vi "Find EXE Root.vi"(10 "Path":path) -> (2 "Location of EXE":path)   [LabVIEW 2026, in "Controller Actor.lvlib" / "Controller.lvclass"]
uses:
  Controller.lvclass
  Controller.lvclass/Controller.ctl
  <userlib>/_OpenG.lib/file/file.llb/Strip Path Extension - String__ogtk.vi
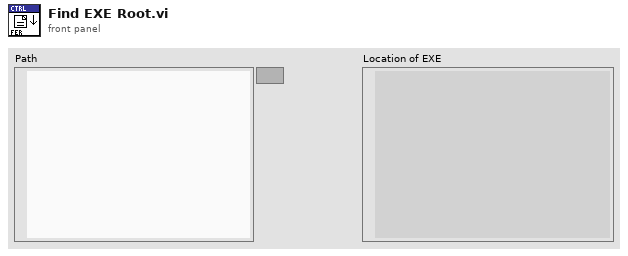
[diagram p1: front panel]
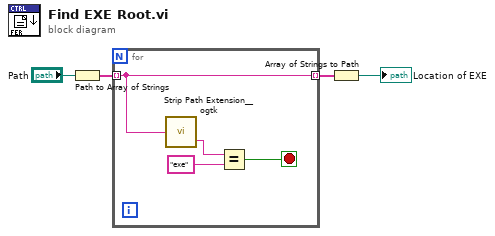
[diagram p0: block diagram]
diagram:
  n1 = Path to Array of Strings(0:"Path") -> (2:w3:string[])  [unwired: 1 out]
  n2 = for {
    tunnel: w3 -> [w8] mode=indexing
    tunnel: [w8] -> w2 mode=indexing
    stop <- w7 stop-if-true
    n3 = call-poly <userlib>:"Strip Path Extension__ogtk.vi"("path"=w8) -> ("extension"=w6:string)  [unwired: 1 out]
    n4 = Equal?(x=w6, y="exe") -> (x = y?=w7:bool)
  }
  n5 = Array of Strings to Path(0:w2) -> (2:→"Location of EXE":path)  [unwired: 1 in]
